vi "FieldCentricTargetAngle.vi"(1 "Dist. From Target[in.] in":dbl, 2 "Width(px)":dbl) -> (0 "Angle of Target":dbl)   [LabVIEW 2019]
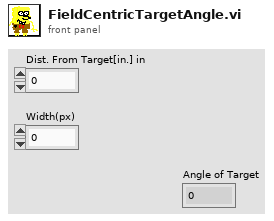
[diagram p1: front panel]
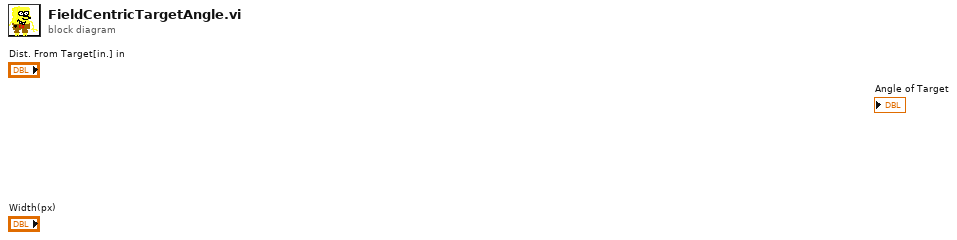
[diagram p0: block diagram]
diagram:
